vi "Power Accuracy Append Group Data Fields.vi"(10 "Power Accuracy Results":T1={"Measurement Cycles"=0, "Measurement Data"=[], "Pass?"=FALSE, "Instruments to Use"={"PIM Instrument Record"={"ixInstrument"=0, "sxInstrumentId"="", "sDriverId"="", "sDriverType"="", "sSerialNumber"="", "tLastCalibration"=timestamp(0 s since 1904-01-01), "tCalibrationDue"=timestamp(0 s since 1904-01-01), "sConfiguration"=""}, "PWM Instrument Record"={"ixInstrument"=0, "sxInstrumentId"="", "sDriverId"="", "sDriverType"="", "sSerialNumber"="", "tLastCalibration"=timestamp(0 s since 1904-01-01), "tCalibrationDue"=timestamp(0 s since 1904-01-01), "sConfiguration"=""}}, "Power Accuracy Test Parameters"={"Stimulus"={"Power Start"=38, "Power Stop"=46, "Frequency Type"=enum."Band Edges", "Frequency Points"=[], "TX 1 Frequency (MHz)"={"Min"=0.0, "Max"=0.0}, "TX 2 Frequency (MHz)"={"Min"=0.0, "Max"=0.0}, "RX Frequency (MHz)"={"Min"=0.0, "Max"=0.0}, "Pad Model Number"="", "Pad Serial Number"="", "Pad Values"=[]}, "Measurement"={"DUT Port"=enum."Port 1", "Direction"=0}, "Display"={"Power"={"Min"=-160, "Max"=-60}, "Tolerance"={"Min"=0.0, "Max"=0.0}}, "Limit"={"Tolerance"=0.35}, "Calibration"={"Calibrated?"=FALSE}}, "Calculated Values"={"C1 Measured Error Min (dB)"=0.0, "C1 Measured Error Max (dB)"=0.0, "C1 Requested Error Min (dB)"=0.0, "C1 Requested Error Max (dB)"=0.0, "C2 Measured Error Min (dB)"=0.0, "C2 Measured Error Max (dB)"=0.0, "C2 Requested Error Min (dB)"=0.0, "C2 Requested Error Max (dB)"=0.0}} {"Power Accuracy Test Parameters"."Measurement"."Direction" items=["Reverse", "Forward", "Auxiliary"]}, 11 "Fields In":T13[](array[typedef])) -> (3 "Fields Out":T13[](array[typedef]))   [LabVIEW 2011]
uses:
  server/database/Fields/Field Record.ctl
  server/database/Fields/Field DataTypes.ctl
  server/database/Fields/Field NextItem.ctl
  TypeDefs/Power Accuracy Results.ctl
  TypeDefs/Power Accuracy Measurement Data.ctl
  server/database/Stations/Instruments/Instrument Record.ctl
  TypeDefs/Power Accuracy Test Parameters.ctl
  TypeDefs/Power Accuracy Stimulus Parameters.ctl
  TypeDefs/Power Accuracy Measurement Parameters.ctl
  BPIMCore EXT/HW IO/DUTport.ctl
  BPIMCore EXT/HW IO/MeasMode.ctl
  TypeDefs/Power Accuracy Display Parameters.ctl
  TypeDefs/Power Accuracy Limit Parameters.ctl
  TypeDefs/Power Accuracy Calibration State.ctl
  TypeDefs/Power Accuracy Calculated Values.ctl
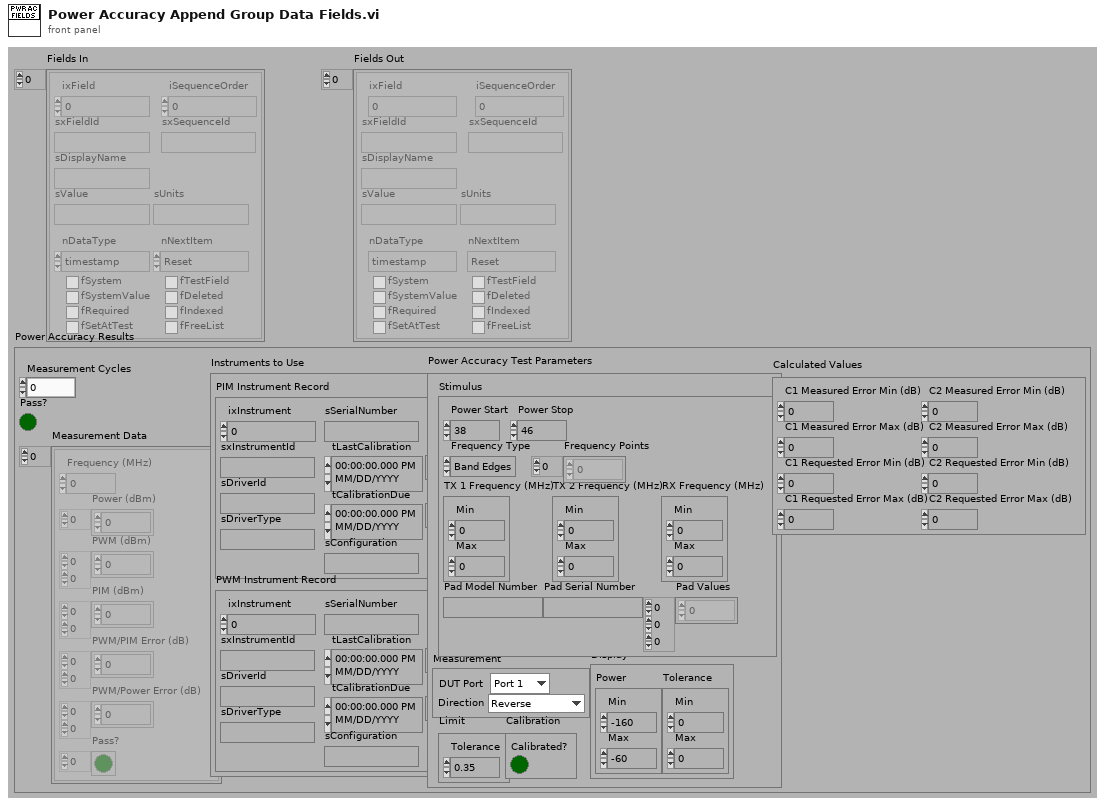
[diagram p1: front panel]
types:
  T1 = typedef "Power Accuracy Results.ctl" = cluster{"Measurement Cycles":i32, "Measurement Data":T2[], "Pass?":bool, "Instruments to Use":cluster{"PIM Instrument Record":T3, "PWM Instrument Record":T3}, "Power Accuracy Test Parameters":T4, "Calculated Values":T12}
  T2 = typedef "Power Accuracy Measurement Data.ctl" = cluster{"Frequency (MHz)":dbl, "Power (dBm)":i32[], "PWM (dBm)":dbl[][], "PIM (dBm)":dbl[][], "PWM/PIM Error (dB)":dbl[][], "PWM/Power Error (dB)":dbl[][], "Pass?":bool[]}
  T3 = typedef "Instrument Record.ctl" = cluster{"ixInstrument":i32, "sxInstrumentId":string, "sDriverId":string, "sDriverType":string, "sSerialNumber":string, "tLastCalibration":timestamp, "tCalibrationDue":timestamp, "sConfiguration":string}
  T4 = typedef "Power Accuracy Test Parameters.ctl" = cluster{"Stimulus":T5, "Measurement":T6, "Display":T9, "Limit":T10, "Calibration":T11}
  T5 = typedef "Power Accuracy Stimulus Parameters.ctl" = cluster{"Power Start":i32, "Power Stop":i32, "Frequency Type":enum16{"Band Edges", "Custom"}, "Frequency Points":dbl[], "TX 1 Frequency (MHz)":cluster{"Min":dbl, "Max":dbl}, "TX 2 Frequency (MHz)":cluster{"Min":dbl, "Max":dbl}, "RX Frequency (MHz)":cluster{"Min":dbl, "Max":dbl}, "Pad Model Number":string, "Pad Serial Number":string, "Pad Values":dbl[][][]}
  T6 = typedef "Power Accuracy Measurement Parameters.ctl" = cluster{"DUT Port":T7, "Direction":T8}
  T7 = typedef "DUTport.ctl" = enum16{"Port 1", "Port 2"}
  T8 = typedef "MeasMode.ctl" = u16
  T9 = typedef "Power Accuracy Display Parameters.ctl" = cluster{"Power":cluster{"Min":i32, "Max":i32}, "Tolerance":cluster{"Min":dbl, "Max":dbl}}
  T10 = typedef "Power Accuracy Limit Parameters.ctl" = cluster{"Tolerance":dbl}
  T11 = typedef "Power Accuracy Calibration State.ctl" = cluster{"Calibrated?":bool}
  T12 = typedef "Power Accuracy Calculated Values.ctl" = cluster{"C1 Measured Error Min (dB)":dbl, "C1 Measured Error Max (dB)":dbl, "C1 Requested Error Min (dB)":dbl, "C1 Requested Error Max (dB)":dbl, "C2 Measured Error Min (dB)":dbl, "C2 Measured Error Max (dB)":dbl, "C2 Requested Error Min (dB)":dbl, "C2 Requested Error Max (dB)":dbl}
  T13 = typedef "Field Record.ctl" = cluster{"ixField":i32, "iSequenceOrder":i32, "sxFieldId":string, "sxSequenceId":string, "sDisplayName":string, "sValue":string, "sUnits":string, "nDataType":T14, "nNextItem":T15, "fSystem":bool, "fSystemValue":bool, "fRequired":bool, "fSetAtTest":bool, "fTestField":bool, "fDeleted":bool, "fIndexed":bool, "fFreeList":bool}
  T14 = typedef "Field DataTypes.ctl" = enum32{"text", "numeric", "list", "timestamp", "boolean"}
  T15 = typedef "Field NextItem.ctl" = enum32{"Reset", "Retain", "Auto-Increment"}
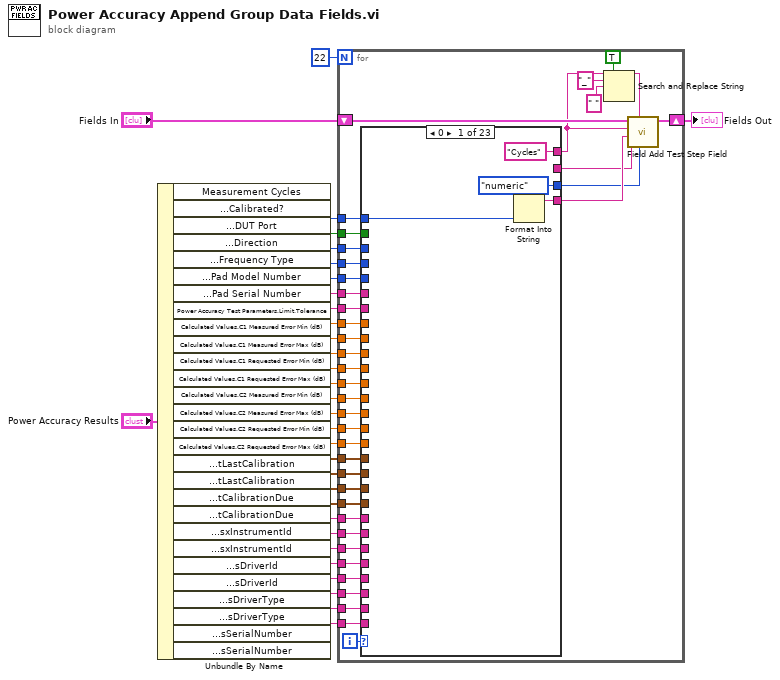
[diagram p0: block diagram]
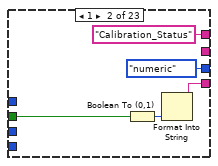
[diagram p2: hidden frame]
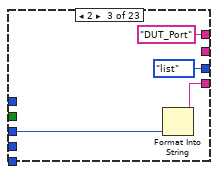
[diagram p3: hidden frame]
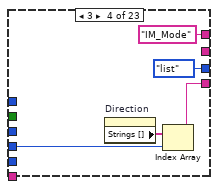
[diagram p4: hidden frame]
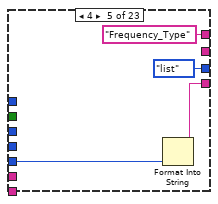
[diagram p5: hidden frame]
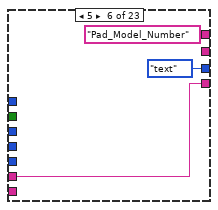
[diagram p6: hidden frame]
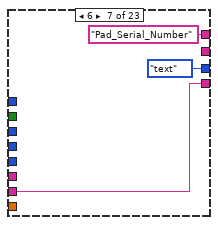
[diagram p7: hidden frame]
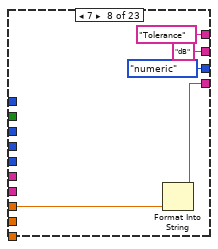
[diagram p8: hidden frame]
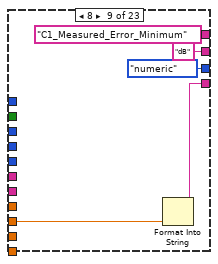
[diagram p9: hidden frame]
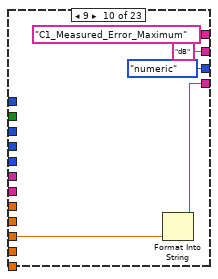
[diagram p10: hidden frame]
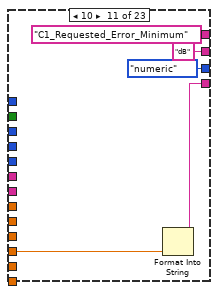
[diagram p11: hidden frame]
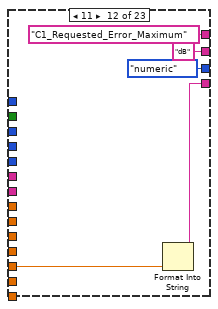
[diagram p12: hidden frame]
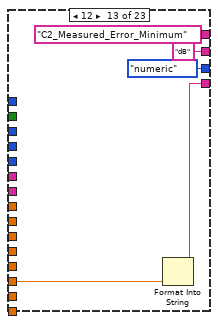
[diagram p13: hidden frame]
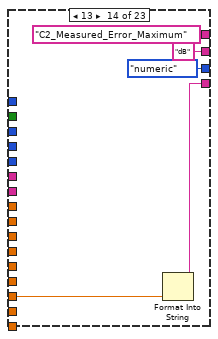
[diagram p14: hidden frame]
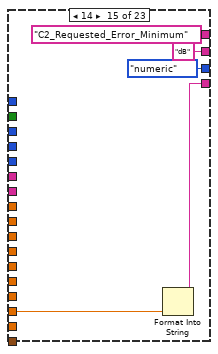
[diagram p15: hidden frame]
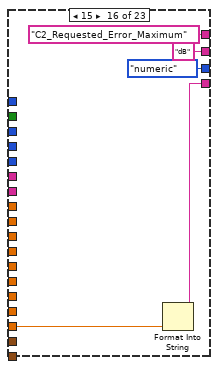
[diagram p16: hidden frame]
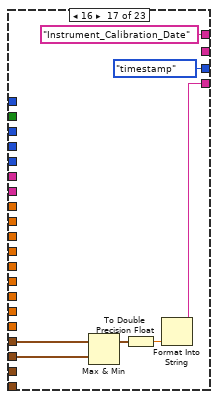
[diagram p17: hidden frame]
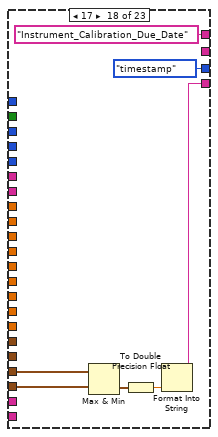
[diagram p18: hidden frame]
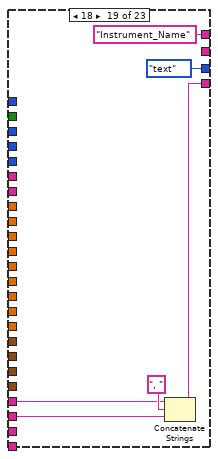
[diagram p19: hidden frame]
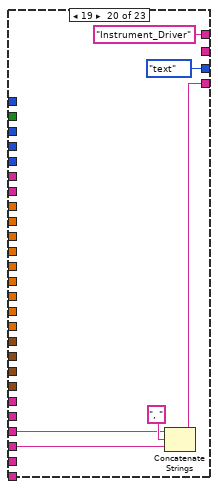
[diagram p20: hidden frame]
diagram:
  n1 = Unbundle By Name("Power Accuracy Results") -> ("Measurement Cycles"=w28:i32, "Power Accuracy Test Parameters.Calibration.Calibrated?"=w27:bool, "Power Accuracy Test Parameters.Measurement.DUT Port"=w26:T7, "Power Accuracy Test Parameters.Measurement.Direction"=w18:T8, "Power Accuracy Test Parameters.Stimulus.Frequency Type"=w19:enum16{"Band Edges", "Custom"}, "Power Accuracy Test Parameters.Stimulus.Pad Model Number"=w11:string, "Power Accuracy Test Parameters.Stimulus.Pad Serial Number"=w10:string, "Power Accuracy Test Parameters.Limit.Tolerance"=w9:dbl, "Calculated Values.C1 Measured Error Min (dB)"=w8:dbl, "Calculated Values.C1 Measured Error Max (dB)"=w7:dbl, "Calculated Values.C1 Requested Error Min (dB)"=w6:dbl, "Calculated Values.C1 Requested Error Max (dB)"=w5:dbl, "Calculated Values.C2 Measured Error Min (dB)"=w4:dbl, "Calculated Values.C2 Measured Error Max (dB)"=w3:dbl, "Calculated Values.C2 Requested Error Min (dB)"=w2:dbl, "Calculated Values.C2 Requested Error Max (dB)"=w1:dbl, "Instruments to Use.PIM Instrument Record.tLastCalibration"=w25:timestamp, "Instruments to Use.PWM Instrument Record.tLastCalibration"=w12:timestamp, "Instruments to Use.PIM Instrument Record.tCalibrationDue"=w24:timestamp, "Instruments to Use.PWM Instrument Record.tCalibrationDue"=w13:timestamp, "Instruments to Use.PIM Instrument Record.sxInstrumentId"=w23:string, "Instruments to Use.PWM Instrument Record.sxInstrumentId"=w17:string, "Instruments to Use.PIM Instrument Record.sDriverId"=w22:string, "Instruments to Use.PWM Instrument Record.sDriverId"=w16:string, "Instruments to Use.PIM Instrument Record.sDriverType"=w21:string, "Instruments to Use.PWM Instrument Record.sDriverType"=w15:string, "Instruments to Use.PIM Instrument Record.sSerialNumber"=w20:string, "Instruments to Use.PWM Instrument Record.sSerialNumber"=w14:string)
  n2 = for {
    N: 22 -> [_]
    shift-right: [w69] -> w31
    shift-left: "Fields In" -> [w70]
    tunnel: w28 -> [w65]
    tunnel: w27 -> [w64]
    tunnel: w26 -> [w63]
    tunnel: w25 -> [w62]
    tunnel: w24 -> [w61]
    tunnel: w23 -> [w60]
    tunnel: w22 -> [w59]
    tunnel: w21 -> [w58]
    tunnel: w20 -> [w57]
    tunnel: w19 -> [w56]
    tunnel: w18 -> [w50]
    tunnel: w17 -> [w49]
    tunnel: w16 -> [w48]
    tunnel: w15 -> [w47]
    tunnel: w14 -> [w46]
    tunnel: w13 -> [w45]
    tunnel: w12 -> [w44]
    tunnel: w11 -> [w43]
    tunnel: w10 -> [w42]
    tunnel: w9 -> [w41]
    tunnel: w8 -> [w40]
    tunnel: w7 -> [w39]
    tunnel: w6 -> [w38]
    tunnel: w5 -> [w37]
    tunnel: w4 -> [w36]
    tunnel: w3 -> [w35]
    tunnel: w2 -> [w34]
    tunnel: w1 -> [w33]
    i -> [w71]
    n3 = case shown="0" w71 {
      tunnel: ["Cycles" ("Field_ID") "Calibration_Status" ("Field_ID") "DUT_Port" ("Field_ID") "IM_Mode" ("Field_ID") "Frequency_Type" ("Field_ID") "Pad_Model_Number" ("Field_ID") "Pad_Serial_Number" ("Field_ID") "Tolerance" ("Field_ID") "C1_Measured_Error_Minimum" ("Field_ID") "C1_Measured_Error_Maximum" ("Field_ID") "C1_Requested_Error_Minimum" ("Field_ID") "C1_Requested_Error_Maximum" ("Field_ID") "C2_Measured_Error_Minimum" ("Field_ID") "C2_Measured_Error_Maximum" ("Field_ID") "C2_Requested_Error_Minimum" ("Field_ID") "C2_Requested_Error_Maximum" ("Field_ID") "Instrument_Calibration_Date" ("Field_ID") "Instrument_Calibration_Due_Date" ("Field_ID") "Instrument_Name" ("Field_ID") "Instrument_Driver" ("Field_ID") "Instrument_Type" ("Field_ID") "Instrument_Serial_Number" ("Field_ID") _] -> w52
      tunnel: [Field_DataTypes."numeric" ("Data Type") Field_DataTypes."numeric" ("Data Type") Field_DataTypes."list" ("Data Type") Field_DataTypes."list" ("Data Type") Field_DataTypes."list" ("Data Type") Field_DataTypes."text" ("Data Type") Field_DataTypes."text" ("Data Type") Field_DataTypes."numeric" ("Data Type") Field_DataTypes."numeric" ("Data Type") Field_DataTypes."numeric" ("Data Type") Field_DataTypes."numeric" ("Data Type") Field_DataTypes."numeric" ("Data Type") Field_DataTypes."numeric" ("Data Type") Field_DataTypes."numeric" ("Data Type") Field_DataTypes."numeric" ("Data Type") Field_DataTypes."numeric" ("Data Type") Field_DataTypes."timestamp" ("Data Type") Field_DataTypes."timestamp" ("Data Type") Field_DataTypes."text" ("Data Type") Field_DataTypes."text" ("Data Type") Field_DataTypes."text" ("Data Type") Field_DataTypes."text" ("Data Type") Field_DataTypes."text" ("Data Type")] -> w67
      tunnel: [w74 w79 w83 w86 w91 w94 w97 w102 w107 w112 w117 w122 w127 w132 w137 w142 w147 w152 w160 w165 w172 w179 _] -> w68
      tunnel: [_ _ _ _ _ _ _ "dB" "dB" "dB" "dB" "dB" "dB" "dB" "dB" "dB" _ _ _ _ _ _ ""] -> w66
      tunnel: w65 -> [w72 _ _ _ _ _ _ _ _ _ _ _ _ _ _ _ _ _ _ _ _ _ _]
      tunnel: w64 -> [_ w77 _ _ _ _ _ _ _ _ _ _ _ _ _ _ _ _ _ _ _ _ _]
      tunnel: w63 -> [_ _ w81 _ _ _ _ _ _ _ _ _ _ _ _ _ _ _ _ _ _ _ _]
      tunnel: w62 -> [_ _ _ _ _ _ _ _ _ _ _ _ _ _ _ _ w146 _ _ _ _ _ _]
      tunnel: w61 -> [_ _ _ _ _ _ _ _ _ _ _ _ _ _ _ _ _ w154 _ _ _ _ _]
      tunnel: w60 -> [_ _ _ _ _ _ _ _ _ _ _ _ _ _ _ _ _ _ w161 _ _ _ _]
      tunnel: w59 -> [_ _ _ _ _ _ _ _ _ _ _ _ _ _ _ _ _ _ _ w167 _ _ _]
      tunnel: w58 -> [_ _ _ _ _ _ _ _ _ _ _ _ _ _ _ _ _ _ _ _ w173 _ _]
      tunnel: w57 -> [_ _ _ _ _ _ _ _ _ _ _ _ _ _ _ _ _ _ _ _ _ w180 _]
      tunnel: w56 -> [_ _ _ _ w90 _ _ _ _ _ _ _ _ _ _ _ _ _ _ _ _ _ _]
      tunnel: w50 -> [_ _ _ w87 _ _ _ _ _ _ _ _ _ _ _ _ _ _ _ _ _ _ _]
      tunnel: w49 -> [_ _ _ _ _ _ _ _ _ _ _ _ _ _ _ _ _ _ w159 _ _ _ _]
      tunnel: w48 -> [_ _ _ _ _ _ _ _ _ _ _ _ _ _ _ _ _ _ _ w166 _ _ _]
      tunnel: w47 -> [_ _ _ _ _ _ _ _ _ _ _ _ _ _ _ _ _ _ _ _ w171 _ _]
      tunnel: w46 -> [_ _ _ _ _ _ _ _ _ _ _ _ _ _ _ _ _ _ _ _ _ w178 _]
      tunnel: w45 -> [_ _ _ _ _ _ _ _ _ _ _ _ _ _ _ _ _ w153 _ _ _ _ _]
      tunnel: w44 -> [_ _ _ _ _ _ _ _ _ _ _ _ _ _ _ _ w145 _ _ _ _ _ _]
      tunnel: w43 -> [_ _ _ _ _ w94 _ _ _ _ _ _ _ _ _ _ _ _ _ _ _ _ _]
      tunnel: w42 -> [_ _ _ _ _ _ w97 _ _ _ _ _ _ _ _ _ _ _ _ _ _ _ _]
      tunnel: w41 -> [_ _ _ _ _ _ _ w101 _ _ _ _ _ _ _ _ _ _ _ _ _ _ _]
      tunnel: w40 -> [_ _ _ _ _ _ _ _ w105 _ _ _ _ _ _ _ _ _ _ _ _ _ _]
      tunnel: w39 -> [_ _ _ _ _ _ _ _ _ w110 _ _ _ _ _ _ _ _ _ _ _ _ _]
      tunnel: w38 -> [_ _ _ _ _ _ _ _ _ _ w115 _ _ _ _ _ _ _ _ _ _ _ _]
      tunnel: w37 -> [_ _ _ _ _ _ _ _ _ _ _ w120 _ _ _ _ _ _ _ _ _ _ _]
      tunnel: w36 -> [_ _ _ _ _ _ _ _ _ _ _ _ w125 _ _ _ _ _ _ _ _ _ _]
      tunnel: w35 -> [_ _ _ _ _ _ _ _ _ _ _ _ _ w130 _ _ _ _ _ _ _ _ _]
      tunnel: w34 -> [_ _ _ _ _ _ _ _ _ _ _ _ _ _ w135 _ _ _ _ _ _ _ _]
      tunnel: w33 -> [_ _ _ _ _ _ _ _ _ _ _ _ _ _ _ w140 _ _ _ _ _ _ _]
      frame 0 {
        n4 = Format Into String(w72) -> (resulting string=w74:string)  [unwired: 3 in, 1 out]
      }
      frame 1 {
        n5 = Boolean To (0,1)(Boolean=w77) -> (0, 1=w76:i16)
        n6 = Format Into String(w76) -> (resulting string=w79:string)  [unwired: 3 in, 1 out]
      }
      frame 2 {
        n7 = Format Into String(w81) -> (resulting string=w83:string)  [unwired: 3 in, 1 out]
      }
      frame 3 {
        n8 = property on="Direction" class="Ring (strict)"() -> ("Strings []"=w85:string[])  [unwired: 2 in, 2 out]
        n9 = Index Array(array=w85, index=w87) -> (element=w86:string)
      }
      frame 4 {
        n10 = Format Into String(w90) -> (resulting string=w91:string)  [unwired: 3 in, 1 out]
      }
      frame 5 {
      }
      frame 6 {
      }
      frame 7 {
        n11 = Format Into String(w101) -> (resulting string=w102:string)  [unwired: 3 in, 1 out]
      }
      frame 8 {
        n12 = Format Into String(w105) -> (resulting string=w107:string)  [unwired: 3 in, 1 out]
      }
      frame 9 {
        n13 = Format Into String(w110) -> (resulting string=w112:string)  [unwired: 3 in, 1 out]
      }
      frame 10 {
        n14 = Format Into String(w115) -> (resulting string=w117:string)  [unwired: 3 in, 1 out]
      }
      frame 11 {
        n15 = Format Into String(w120) -> (resulting string=w122:string)  [unwired: 3 in, 1 out]
      }
      frame 12 {
        n16 = Format Into String(w125) -> (resulting string=w127:string)  [unwired: 3 in, 1 out]
      }
      frame 13 {
        n17 = Format Into String(w130) -> (resulting string=w132:string)  [unwired: 3 in, 1 out]
      }
      frame 14 {
        n18 = Format Into String(w135) -> (resulting string=w137:string)  [unwired: 3 in, 1 out]
      }
      frame 15 {
        n19 = Format Into String(w140) -> (resulting string=w142:string)  [unwired: 3 in, 1 out]
      }
      frame 16 {
        n20 = Max & Min(x=w146, y=w145) -> (max(x,y)=w148:timestamp)  [unwired: 1 out]
        n21 = To Double Precision Float(number=w148) -> (double precision float=w149:dbl)
        n22 = Format Into String(w149) -> (resulting string=w147:string)  [unwired: 3 in, 1 out]
      }
      frame 17 {
        n23 = Max & Min(x=w154, y=w153) -> (min(x,y)=w155:timestamp)  [unwired: 1 out]
        n24 = To Double Precision Float(number=w155) -> (double precision float=w156:dbl)
        n25 = Format Into String(w156) -> (resulting string=w152:string)  [unwired: 3 in, 1 out]
      }
      frame 18 {
        n26 = Concatenate Strings(w161, ", ", w159) -> (w160:string)
      }
      frame 19 {
        n27 = Concatenate Strings(w167, ", ", w166) -> (w165:string)
      }
      frame 20 {
        n28 = Concatenate Strings(w173, ", ", w171) -> (w172:string)
      }
      frame 21 {
        n29 = call <vilib>:"Trim Whitespace.vi"("string"=w180) -> ("trimmed string"=w177:string)  [unwired: 1 in]
        n30 = Concatenate Strings(w177, ", ", w178) -> (w179:string)
      }
      frame Default {
      }
    }
    n31 = Search and Replace String(replace all?=TRUE ("replace all? (F)"), input string=w52, search string="_", replace string=" " ("replace string (\"\")")) -> (result string=w51:string)  [unwired: 1 in, 6 out]
    n32 = call "Field Add Test Step Field.vi"("nDataType"=w67, "sDisplayName"=w51, "sUnits"=w66, "sValue"=w68, "sxFieldId"=w52, "Fields In"=w70) -> ("Fields Out"=w69:T13[])  [unwired: 5 out]
  }
  "Fields Out" <- w31
